vi "Linear_Flow_Ramp_1.vi"(2 "Debug Mode":bool, 3 "Elapsed Time (s)":dbl, 4 "State":enum16{"Edit", "Start", "Run", "End", "Idle"}(ring), 5 "Argument List In":string[](array[string])) -> (0 "Status Out":string, 1 "Argument List Out":string[](array[string]))   [LabVIEW 2011]
panel:
  in  "Flow to Ramp":u16(ring) items=["Flow1"]
  in  "Select":enum32{"Use Rate", "Use Time/End Flow"}(radio)
  in  "End Flow":dbl caption="End Flow\n(sccm)"
  in  "Total Time":dbl caption="Total Time (sec)"
  in  "Ramp Rate":dbl caption="Ramp Rate\n(sccm/sec)"
  in  "Start Flow":dbl caption="Start Flow\n(sccm)"
  in  "Gas":u16(ring) items=["R_Al", "R_As_Liq", "R_AsH3", "R_Fe", "R_Ga", "R_H2", "R_In", "R_N_Dop", "R_N2", "R_P_Dop", "R_P_Liq", "R_PH3"]
  in  "Active":bool
  in  "Run":bool
  in  "Gas_Source":bool caption="Gas Source"
  in  "H2":bool
  in  "Bubbler":bool
  in  "H2_Dilute":bool caption="H2 Dilute"
  in  "Remote":bool
  in  "Cancel":bool
  in  "OK":bool
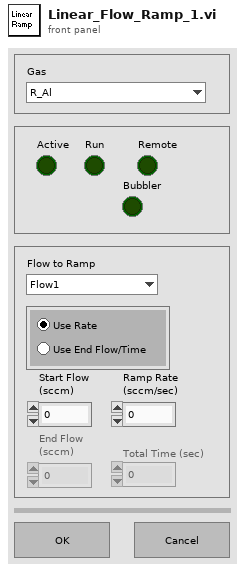
[diagram p1: front panel]
types:
  T1 = enum16{"Discrete", "Continuous", "Instantaneous"}
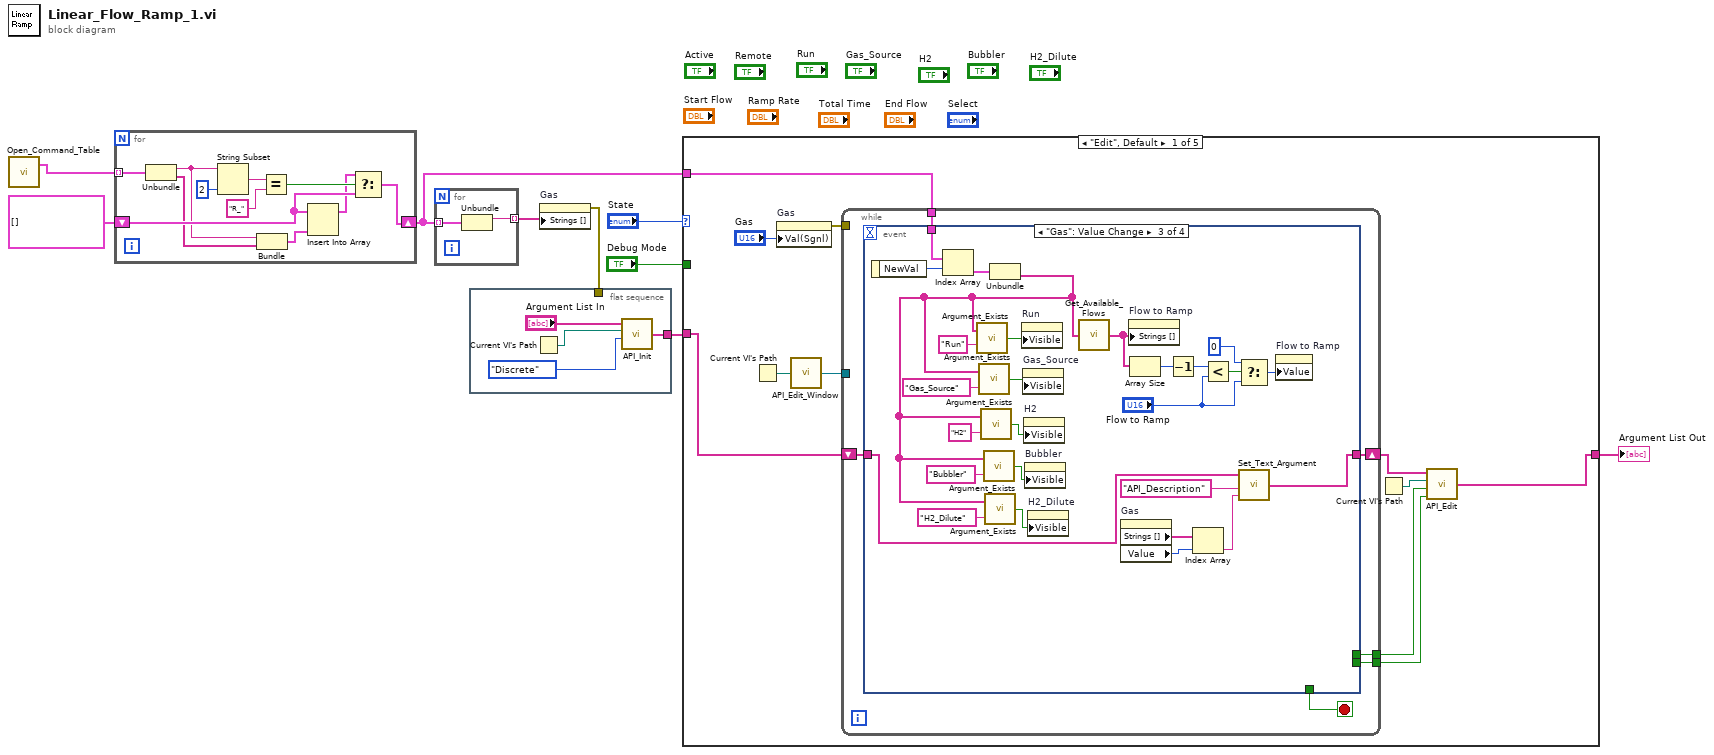
[diagram p0: block diagram]
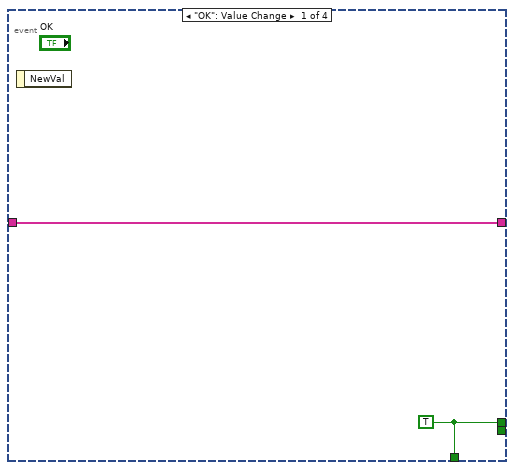
[diagram p2: hidden frame]
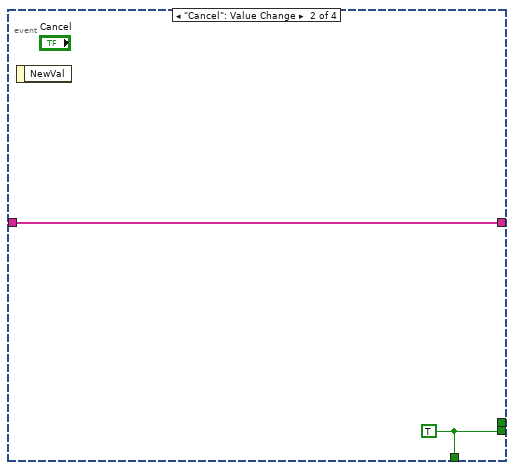
[diagram p3: hidden frame]
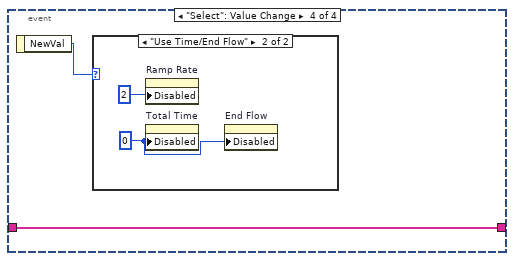
[diagram p4: hidden frame]
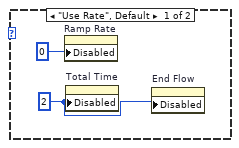
[diagram p5: hidden frame]
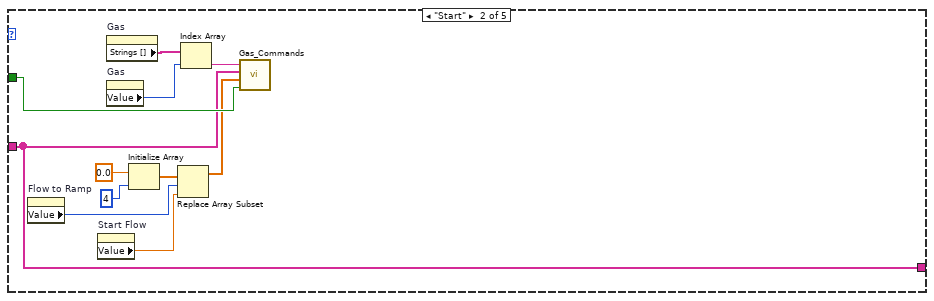
[diagram p6: hidden frame]
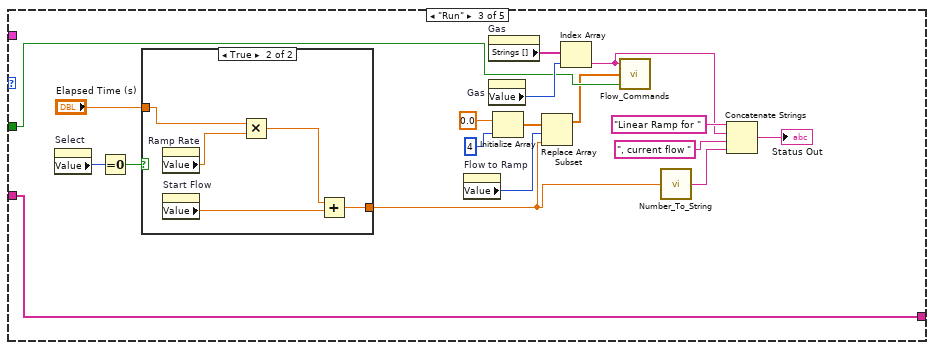
[diagram p7: hidden frame]
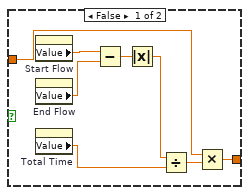
[diagram p8: hidden frame]
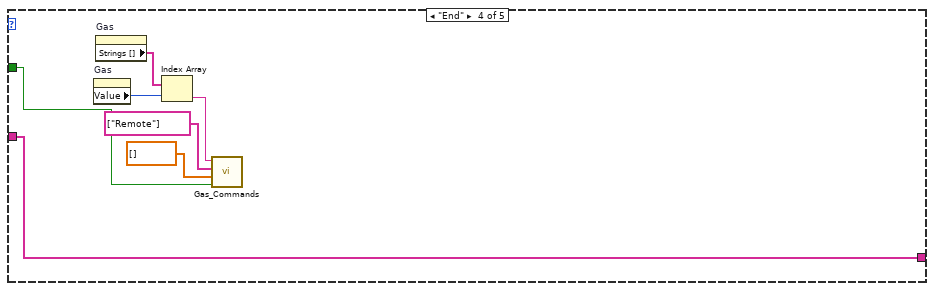
[diagram p9: hidden frame]
diagram:
  n1 = call "Open_Command_Table.vi"() -> ("Commands"=w3:cluster{string, string[]}[])  [unwired: 2 out]
  n2 = for {
    tunnel: w3 -> [w20] mode=indexing
    shift-right: [w15] -> w2
    shift-left: cluster{string, string[]}[] [] ("Commands") -> [w14]
    n3 = Unbundle(w20) -> (w12:string, w11:string[])
    n4 = String Subset(string=w12, length (rest)=2 ("length (rest)")) -> (substring=w18:string)  [unwired: 1 out]
    n5 = Bundle(w12, w11) -> (w10:cluster{string, string[]})  [unwired: 1 out]
    n6 = Equal?(x=w18, y="R_") -> (x = y?=w16:bool)
    n7 = Insert Into Array(array=w14, new element=w10) -> (w13:cluster{string, string[]}[])  [unwired: 1 in]
    n8 = Select(t=w13, s=w16, f=w14) -> (s? t:f=w15:cluster{string, string[]}[])
  }
  n9 = for {
    tunnel: w2 -> [w22] mode=indexing
    tunnel: [w21] -> w5 mode=indexing
    n10 = Unbundle(w22) -> (w21:string)  [unwired: 1 out]
  }
  n11 = flat-sequence {
    tunnel: [w26] -> w6
    tunnel: w1 -> [_]
    frame #0 {
      n12 = Current VI's Path() -> (path=w23:path)
      n13 = call "API_Init.vi"("API Mode"=T1."Discrete", "VI Path"=w23, "Argument List In"="Argument List In") -> ("Argument List Out"=w26:string[])  [unwired: 1 in]
    }
  }
  n14 = property on="Gas" class="Ring (strict)"("Strings []"=w5) -> (error out=w1:errorcluster)  [unwired: 2 in, 1 out]
  n15 = case shown="\"Edit\", Default" "State" {
    tunnel: [w27 w81 w93 w123 w130] -> w8
    tunnel: w6 -> [w28 w81 w93 w123 w130]
    tunnel: "Debug Mode" -> [_ w88 w107 w129 _]
    tunnel: w2 -> [w31 _ _ _ _]
    frame "Edit", Default {
      n16 = Current VI's Path() -> (path=w33:path)
      n17 = property on="Gas" class="Ring (strict)"("Val(Sgnl)"="Gas") -> (error out=w29:errorcluster)  [unwired: 2 in, 1 out]
      n18 = call "API_Edit_Window.vi"("VI Path"=w33) -> ("VI Reference"=w32:refnum<vi>)
      n19 = while {
        tunnel: w31 -> [w42]
        tunnel: [w40] -> w35
        tunnel: [w39] -> w34
        tunnel: w32 -> [_]
        tunnel: w29 -> [_]
        shift-right: [w43] -> w36
        shift-left: w28 -> [w38]
        stop <- w41 stop-if-true
        n20 = event shown="[2] \"Gas\": Value Change" {
          selector: _ -> [_ _ _ _]
          dyn-events: _ -> [_ _ _ _]
          timeout: _ -> [_ _ _ _]
          tunnel: w38 -> [w45 w47 w52 w75]
          tunnel: [w45 w47 w51 w75] -> w43
          tunnel: w42 -> [_ _ w74 _]
          tunnel: [w44 w46 _ _] -> w41
          tunnel: [w44 _ _ _] -> w40
          tunnel: [_ w46 _ _] -> w39
          event "OK": Value Change {
            w44 = TRUE
            n21 = event-data() -> ()  [unwired: 2 out]
          }
          event "Cancel": Value Change {
            w46 = TRUE
            n22 = event-data() -> ()  [unwired: 2 out]
          }
          event "Gas": Value Change {
            n23 = event-data() -> ("NewVal"=w62:u16)  [unwired: 1 out]
            n24 = Index Array(array=w74, index=w62) -> (element=w73:cluster{string, string[]})
            n25 = Unbundle(w73) -> (w57:string[])  [unwired: 1 out]
            n26 = call "Argument_Exists.vi"("Argument"="Run", "Argument List"=w57) -> ("Argument Exists"=w71:bool)
            n27 = call "Argument_Exists.vi"("Argument"="Gas_Source", "Argument List"=w57) -> ("Argument Exists"=w67:bool)
            n28 = call "Argument_Exists.vi"("Argument"="H2", "Argument List"=w57) -> ("Argument Exists"=w68:bool)
            n29 = call "Argument_Exists.vi"("Argument"="Bubbler", "Argument List"=w57) -> ("Argument Exists"=w65:bool)
            n30 = call "Argument_Exists.vi"("Argument"="H2_Dilute", "Argument List"=w57) -> ("Argument Exists"=w63:bool)
            n31 = property on="Run" class="Bool (strict)"("Visible"=w71) -> ()  [unwired: 2 in, 2 out]
            n32 = property on="Gas_Source" class="Bool (strict)"("Visible"=w67) -> ()  [unwired: 2 in, 2 out]
            n33 = property on="H2" class="Bool (strict)"("Visible"=w68) -> ()  [unwired: 2 in, 2 out]
            n34 = property on="Bubbler" class="Bool (strict)"("Visible"=w65) -> ()  [unwired: 2 in, 2 out]
            n35 = property on="H2_Dilute" class="Bool (strict)"("Visible"=w63) -> ()  [unwired: 2 in, 2 out]
            n36 = call "Get_Available_Flows.vi"("Argument List"=w57) -> ("Available Flows"=w55:string[])
            n37 = property on="Gas" class="Ring (strict)"() -> ("Strings []"=w50:string[], "Value"=w49:u16)  [unwired: 2 in, 2 out]
            n38 = property on="Flow to Ramp" class="Ring (strict)"("Strings []"=w55) -> ()  [unwired: 2 in, 2 out]
            n39 = Array Size(array=w55) -> (size(s)=w61:i32)
            n40 = Decrement(x=w61) -> (x-1=w59:i32)
            n41 = Index Array(array=w50, index=w49) -> (element=w48:string)
            n42 = Less?(x=w59, y="Flow to Ramp") -> (x < y?=w60:bool)
            n43 = Select(t=u16 0, s=w60, f="Flow to Ramp") -> (s? t:f=w54:u16)
            n44 = call "Set_Text_Argument.vi"("Text"=w48, "Argument"="API_Description", "Argument List In"=w52) -> ("Argument List Out"=w51:string[])
            n45 = property on="Flow to Ramp" class="Ring (strict)"("Value"=w54) -> ()  [unwired: 2 in, 2 out]
          }
          event "Select": Value Change {
            n46 = event-data() -> ("NewVal"=w76:enum32{"Use Rate", "Use Time/End Flow"})  [unwired: 1 out]
            n47 = case shown="\"Use Time/End Flow\"" w76 {
              frame "Use Rate", Default {
                w77 = u8 2 ("Disabled")
                n48 = property on="Ramp Rate" class="DigNum (strict)"("Disabled"=u8 0) -> ()  [unwired: 2 in, 2 out]
                n49 = property on="Total Time" class="DigNum (strict)"("Disabled"=w77) -> ()  [unwired: 2 in, 2 out]
                n50 = property on="End Flow" class="DigNum (strict)"("Disabled"=w77) -> ()  [unwired: 2 in, 2 out]
              }
              frame "Use Time/End Flow" {
                w79 = u8 0 ("Disabled")
                n51 = property on="Ramp Rate" class="DigNum (strict)"("Disabled"=u8 2) -> ()  [unwired: 2 in, 2 out]
                n52 = property on="Total Time" class="DigNum (strict)"("Disabled"=w79) -> ()  [unwired: 2 in, 2 out]
                n53 = property on="End Flow" class="DigNum (strict)"("Disabled"=w79) -> ()  [unwired: 2 in, 2 out]
              }
            }
          }
        }
      }
      n54 = Current VI's Path() -> (path=w37:path)
      n55 = call "API_Edit.vi"("Cancel"=w34, "OK"=w35, "VI Path"=w37, "Argument List In"=w36) -> ("Argument List Out"=w27:string[])
    }
    frame "Start" {
      n56 = property on="Flow to Ramp" class="Ring (strict)"() -> ("Value"=w85:u16)  [unwired: 2 in, 2 out]
      n57 = property on="Start Flow" class="DigNum (strict)"() -> ("Value"=w83:dbl)  [unwired: 2 in, 2 out]
      n58 = property on="Gas" class="Ring (strict)"() -> ("Strings []"=w91:string[])  [unwired: 2 in, 2 out]
      n59 = property on="Gas" class="Ring (strict)"() -> ("Value"=w90:u16)  [unwired: 2 in, 2 out]
      n60 = Initialize Array(0.0 ("element"), 4 ("dimension size")) -> (w84:dbl[])
      n61 = Replace Array Subset(array=w84, new element=w83, index=w85) -> (w82:dbl[])
      n62 = Index Array(array=w91, index=w90) -> (element=w89:string)
      n63 = call "Gas_Commands.vi"("Debug Mode"=w88, "Flow Array"=w82, "Argument List"=w81, "Command"=w89) -> ()  [unwired: 1 out]
    }
    frame "Run" {
      n64 = property on="Select" class="RadioBtnsControl (strict)"() -> ("Value"=w106:enum32{"Use Rate", "Use Time/End Flow"})  [unwired: 2 in, 2 out]
      n65 = Equal To 0?(x=w106) -> (x = 0?=w92:bool)
      n66 = case shown="True" w92 {
        tunnel: "Elapsed Time (s)" -> [w111 w122]
        tunnel: [w113 w118] -> w96
        frame False {
          n67 = property on="Start Flow" class="DigNum (strict)"() -> ("Value"=w116:dbl)  [unwired: 2 in, 2 out]
          n68 = property on="End Flow" class="DigNum (strict)"() -> ("Value"=w115:dbl)  [unwired: 2 in, 2 out]
          n69 = property on="Total Time" class="DigNum (strict)"() -> ("Value"=w110:dbl)  [unwired: 2 in, 2 out]
          n70 = Subtract(x=w116, y=w115) -> (x-y=w117:dbl)
          n71 = Absolute Value(x=w117) -> (abs(x)=w114:dbl)
          n72 = Divide(x=w114, y=w110) -> (x/y=w112:dbl)
          n73 = Multiply(x=w111, y=w112) -> (x*y=w113:dbl)
        }
        frame True {
          n74 = property on="Ramp Rate" class="DigNum (strict)"() -> ("Value"=w121:dbl)  [unwired: 2 in, 2 out]
          n75 = property on="Start Flow" class="DigNum (strict)"() -> ("Value"=w119:dbl)  [unwired: 2 in, 2 out]
          n76 = Multiply(x=w122, y=w121) -> (x*y=w120:dbl)
          n77 = Add(x=w120, y=w119) -> (x+y=w118:dbl)
        }
      }
      n78 = property on="Flow to Ramp" class="Ring (strict)"() -> ("Value"=w101:u16)  [unwired: 2 in, 2 out]
      n79 = property on="Gas" class="Ring (strict)"() -> ("Strings []"=w109:string[])  [unwired: 2 in, 2 out]
      n80 = property on="Gas" class="Ring (strict)"() -> ("Value"=w108:u16)  [unwired: 2 in, 2 out]
      n81 = Initialize Array(0.0 ("element"), 4 ("dimension size")) -> (w102:dbl[])
      n82 = Replace Array Subset(array=w102, new element=w96, index=w101) -> (w100:dbl[])
      n83 = Index Array(array=w109, index=w108) -> (element=w98:string)
      n84 = call "Flow_Commands.vi"("Debug Mode"=w107, "Flow Array"=w100, "Command"=w98) -> ()  [unwired: 1 out]
      n85 = call "Number_To_String.vi"("Number"=w96) -> ("String"=w95:string)
      n86 = Concatenate Strings("Linear Ramp for " ("string"), w98, ", current flow " ("string"), w95) -> (→"Status Out":string)
    }
    frame "End" {
      n87 = property on="Gas" class="Ring (strict)"() -> ("Value"=w127:u16)  [unwired: 2 in, 2 out]
      n88 = property on="Gas" class="Ring (strict)"() -> ("Strings []"=w128:string[])  [unwired: 2 in, 2 out]
      n89 = Index Array(array=w128, index=w127) -> (element=w126:string)
      n90 = call "Gas_Commands.vi"("Debug Mode"=w129, "Flow Array"=dbl[] [], "Argument List"=string[] ["Remote"], "Command"=w126) -> ()  [unwired: 1 out]
    }
    frame "Idle" {
    }
  }
  "Argument List Out" <- w8
